vi "PTC-Config.vi"(0 "Speaker":string, 5 "Probe mic":string, 7 "Cal mic":string, 9 "Stimulus":T1, 11 "error in (no error)":errorcluster) -> (12 "df (Hz)":dbl, 13 "dt (ms)":dbl, 14 "Mic Avg":dbl[][](array[numeric]), 15 "error out":errorcluster)   [LabVIEW 2020]
uses:
  Common VIs/Typedefs/CAL-Stimulus.ctl
  3c1deb76-fac1-43ef-8724-a3afa18a8211.vi
  2e66f2f8-1149-4e52-90ee-ea76ca7b7918.vi
  epl-vi-lib/PXI DAQ VIs/AODO/AODO-Engine.vi
  epl-vi-lib/PXI DAQ VIs/AIDI/AIDI-Engine.vi
panel:
  out "Stimulus 2":dbl[](array[numeric])
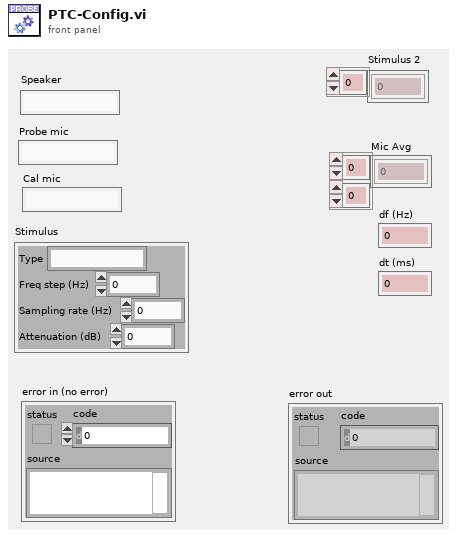
[diagram p1: front panel]
types:
  T1 = typedef "CAL-Stimulus.ctl" = cluster{"Type":string, "Freq step (Hz)":dbl, "Sampling rate (Hz)":dbl, "Attenuation (dB)":dbl}
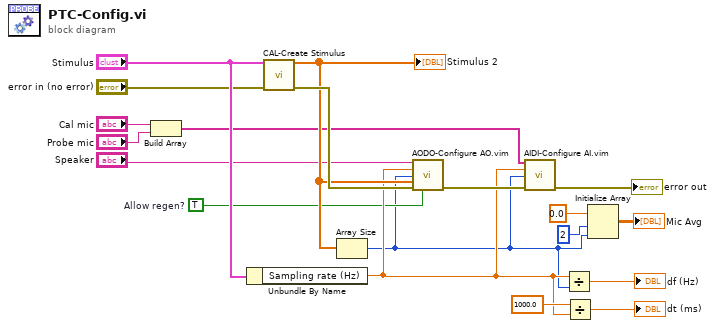
[diagram p0: block diagram]
diagram:
  w7 = TRUE  # Allow regen?
  n1 = Build Array("Cal mic", "Probe mic") -> (w3:string[])
  n2 = Unbundle By Name("Stimulus") -> ("Sampling rate (Hz)"=w9:dbl)
  n3 = call "CAL-Create Stimulus.vi"("Cal Stimulus"="Stimulus", "error in (no error)"="error in (no error)") -> ("Stimulus"=w11:dbl[], "error out"=w12:errorcluster)  [unwired: 12 in]
  "Stimulus 2" <- w11
  n4 = Array Size(array=w11) -> (size(s)=w2:i32)
  n5 = call "AODO-Configure AO.vim"("AO.Channels"="Speaker", "AO.Fs (Hz)"=w9, "AO.Npts"=w2, "AO"=w11, "error in (no error)"=w12, "Allow regen?"=w7) -> ("error out"=w10:errorcluster)  [unwired: 9 in]
  n6 = call "AIDI-Configure AI.vim"("AI.Channels"=w3, "AI.Fs (Hz)"=w9, "AI.Npts"=w2, "error in (no error)"=w10) -> ("error out"=→"error out":errorcluster)  [unwired: 11 in]
  n7 = Divide(x=w9, y=w2) -> (x/y=→"df (Hz)":dbl)
  n8 = Divide(x=1000.0, y=w9) -> (x/y=→"dt (ms)":dbl)
  n9 = Initialize Array(0.0 ("element"), 2 ("dimension size"), w2) -> (→"Mic Avg":dbl[][])
